vi "Init.vi"(0 "STOMP in":refnum<class "STOMP.lvclass">, 5 "error in (no error)":errorcluster) -> (14 "STOMP out":refnum<class "STOMP.lvclass">, 19 "error out":errorcluster)   [LabVIEW 2017, in "LabVIEW STOMP.lvlib" / "STOMP.lvclass"]
uses:
  STOMP.lvclass
  Typedefs/Type_ServerFrame.ctl
  Typedefs/Type_ServerFrameType.ctl
  STOMP.lvclass/STOMP.ctl
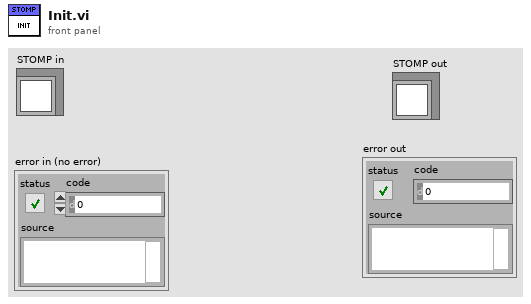
[diagram p1: front panel]
types:
  T1 = typedef "LabVIEW STOMP.lvlib/STOMP.lvclass/Type_ServerFrame.ctl" = cluster{"Type":T2, "Headers":cluster{"Header":string, "Value":string}[], "Body":string}
  T2 = typedef "LabVIEW STOMP.lvlib/STOMP.lvclass/Type_ServerFrameType.ctl" = enum16{"Undefined", "MESSAGE", "CONNECTED", "RECEIPT", "ERROR"}
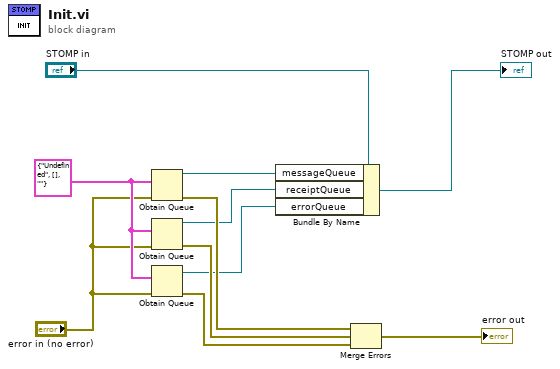
[diagram p0: block diagram]
diagram:
  w7 = T1 {"Type"=enum."Undefined", "Headers"=[], "Body"=""} ("Type_ServerFrame")
  n1 = Obtain Queue(element data type=w7, error in (no error)="error in (no error)") -> (queue out=w10:refnum<queue>, error out=w9:errorcluster)  [unwired: 3 in, 1 out]
  n2 = Obtain Queue(element data type=w7, error in (no error)="error in (no error)") -> (queue out=w2:refnum<queue>, error out=w4:errorcluster)  [unwired: 3 in, 1 out]
  n3 = Obtain Queue(element data type=w7, error in (no error)="error in (no error)") -> (queue out=w1:refnum<queue>, error out=w3:errorcluster)  [unwired: 3 in, 1 out]
  n4 = Bundle By Name(cluster="STOMP in", "messageQueue"=w10, "receiptQueue"=w2, "errorQueue"=w1) -> (→"STOMP out":refnum<class "STOMP.lvclass">)
  n5 = Merge Errors(w9, w4, w3) -> (→"error out":errorcluster)
